vi "NiFPGA Close.vi"(7 "Attribute":T1(ring), 8 "error in (no error)":errorcluster, 11 "Session":u32) -> (0 "error out":errorcluster, 2 "Status":i32, 3 "Session Out":u32)   [LabVIEW 2011, in "Scan Engine Custom Device.lvlib"]
doc: "Closes the session to the FPGA. The FPGA resets unless either another session is still open or you use the NiFpga_CloseAttribute_NoResetIfLastSession attribute."
uses:
  Scan Engine Custom Device.lvlib
  NiFpga.dll
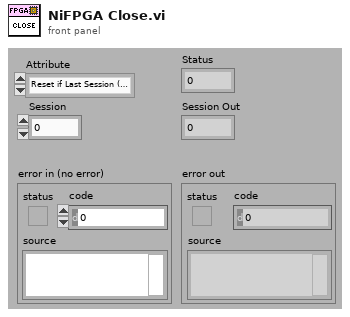
[diagram p1: front panel]
types:
  T1 = enum32{"Reset if Last Session (Default)", "No Reset"}
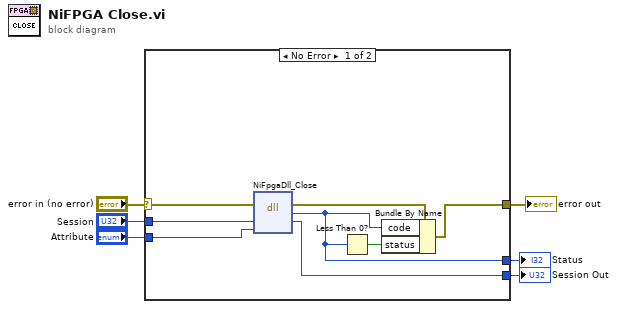
[diagram p0: block diagram]
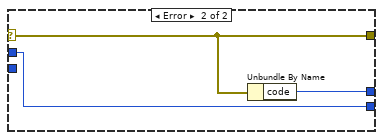
[diagram p2: hidden frame]
diagram:
  n1 = case shown="No Error" "error in (no error)" {
    selector: "error in (no error)" -> [w14 w16]
    tunnel: [w10 w16] -> w5
    tunnel: "Session" -> [w13 w17]
    tunnel: [w12 w17] -> w3
    tunnel: [w8 w15] -> w2
    tunnel: "Attribute" -> [w7 _]
    frame No Error {
      n2 = dll-call lib="NiFpga.dll" fn="NiFpgaDll_Close"(error in=w14, "Session"=w13, "Attribute"=w7) -> (error out=w11:errorcluster, "Status"=w8:i32, "Session"=w12:u32)  [unwired: 3 in, 1 out]
      n3 = Less Than 0?(x=w8) -> (x < 0?=w9:bool)
      n4 = Bundle By Name(cluster=w11, "code"=w8, "status"=w9) -> (w10:errorcluster)
    }
    frame Error {
      n5 = Unbundle By Name(w16) -> ("code"=w15:i32)
    }
  }
  "error out" <- w5
  "Session Out" <- w3
  "Status" <- w2
